vi "OAuth2 Error Message.vi"(5 "Redirect URI":refnum<class "URI.lvclass">, 7 "Requested Scopes":string[](array[string]), 10 "OAuth2 Error":T1, 11 "error_description":string) -> (2 "Error Message":string, 3 "Error Code":i32)   [LabVIEW 2020, in "OAuth2.lvlib"]
uses:
  OAuth2.lvlib
  OAuth2 Error.ctl
  <vilib>/IlluminatedG/lv-stream/URI/URI.lvclass
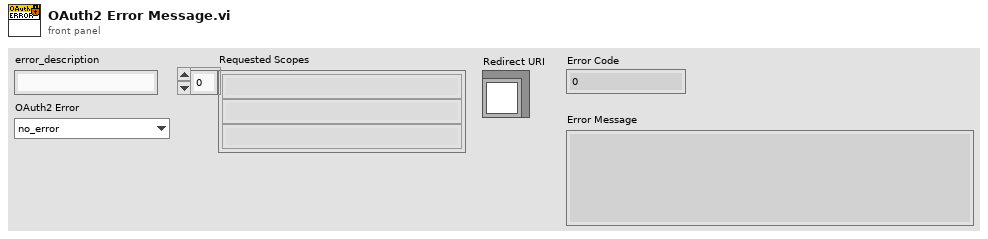
[diagram p1: front panel]
types:
  T1 = typedef "OAuth2.lvlib/OAuth2 Error.ctl" = enum16{"no_error", "admin_policy_enforced", "disallowed_useragent", "org_internal", "invalid_grant", "redirect_uri_mismatch", "invalid_request", "access_denied"}
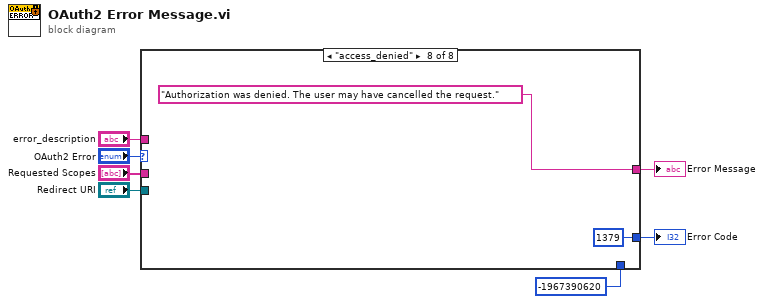
[diagram p0: block diagram]
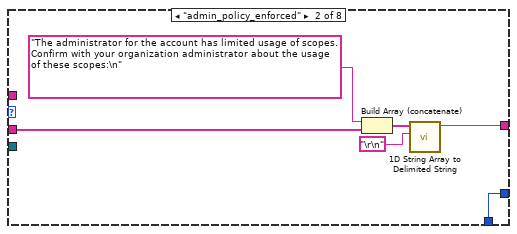
[diagram p3: hidden frame]
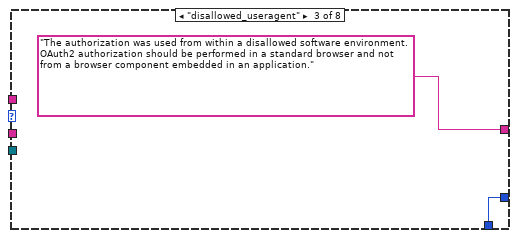
[diagram p4: hidden frame]
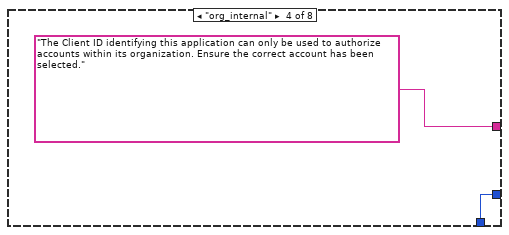
[diagram p5: hidden frame]
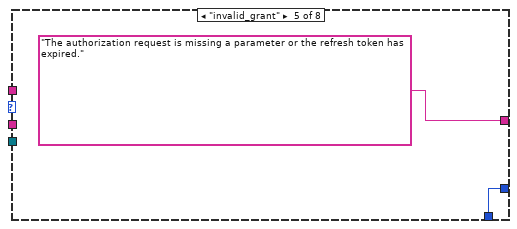
[diagram p6: hidden frame]
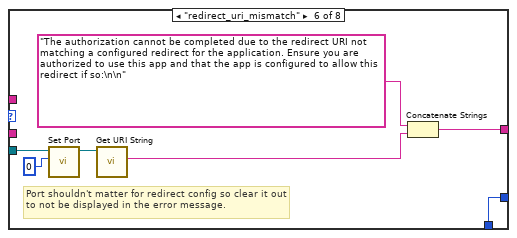
[diagram p7: hidden frame]
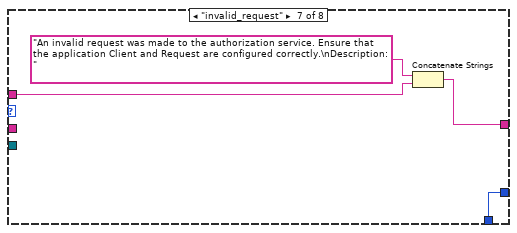
[diagram p8: hidden frame]
diagram:
  n1 = case shown="\"access_denied\"" "OAuth2 Error" {
    tunnel: "Requested Scopes" -> [_ w14 _ _ _ _ _ _]
    tunnel: [_ w10 "The authorization was used from within a disallowed software environment. OAuth2 authorization should be performed in a standard browser and not from a browser component embedded in an application." "The Client ID identifying this application can only be used to authorize accounts within its organization. Ensure the correct account has been selected." "The authorization request is missing a parameter or the refresh token has expired." w22 w29 "Authorization was denied. The user may have cancelled the request."] -> w5
    tunnel: "Redirect URI" -> [_ _ _ _ _ w27 _ _]
    tunnel: "error_description" -> [_ _ _ _ _ _ w31 _]
    tunnel: -1967390620 -> [w8 w9 w15 w17 w19 w21 w28 _]
    tunnel: [w8 w9 w15 w17 w19 w21 w28 1379] -> w1
    frame "no_error" {
    }
    frame "admin_policy_enforced" {
      n2 = Build Array (concatenate)("The administrator for the account has limited usage of scopes. Confirm with your organization administrator about the usage of these scopes:\n", w14) -> (w12:string[])
      n3 = call <vilib>:"1D String Array to Delimited String.vi"("delimiter"="\r\n", "string array"=w12) -> ("delimited string"=w10:string)  [unwired: 9 in]
    }
    frame "disallowed_useragent" {
    }
    frame "org_internal" {
    }
    frame "invalid_grant" {
    }
    frame "redirect_uri_mismatch" {
      # "Port shouldn't matter for redirect config so clear it out to not be displayed in the error message."
      n4 = call <vilib>:"Set Port.vi"("Port"=u16 0, "URI in"=w27) -> ("URI out"=w25:refnum<class "URI.lvclass">)  [unwired: 8 in, 1 out]
      n5 = call <vilib>:"Get URI String.vi"("URI in"=w25) -> ("URI String"=w23:string)  [unwired: 8 in, 2 out]
      n6 = Concatenate Strings("The authorization cannot be completed due to the redirect URI not matching a configured redirect for the application. Ensure you are authorized to use this app and that the app is configured to allow this redirect if so:\n\n", w23) -> (w22:string)
    }
    frame "invalid_request" {
      n7 = Concatenate Strings("An invalid request was made to the authorization service. Ensure that the application Client and Request are configured correctly.\nDescription: ", w31) -> (w29:string)
    }
    frame "access_denied" {
    }
  }
  "Error Message" <- w5
  "Error Code" <- w1
